vi "StartOnDemandAcquisitionRoutedMessage_Parse.vi"(8 "error in (no error)":errorcluster, 11 "message":variant) -> (0 "error out":errorcluster, 2 "on demand acq config":T1)   [LabVIEW 2017, in "EmsaAcquisition.lvlib"]
uses:
  <vilib>/addons/InsightCM/Devices/Shared/Emsa/EmsaAcquisition/EmsaAcquisition.lvlib
  <vilib>/addons/InsightCM/Devices/Shared/Emsa/EmsaAcquisition/controls/StartOnDemandAcquisitionRoutedMessage.ctl
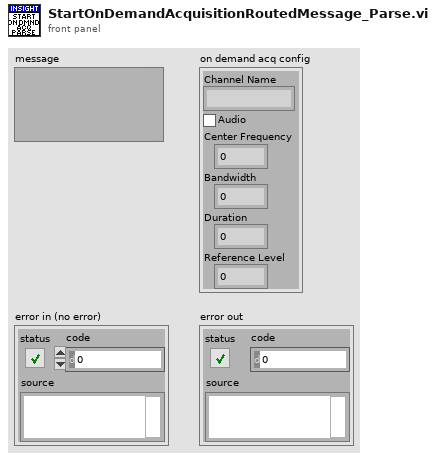
[diagram p1: front panel]
types:
  T1 = typedef "EmsaAcquisition.lvlib/StartOnDemandAcquisitionRoutedMessage.ctl" = cluster{"Channel Name":string, "Audio":bool, "Center Frequency":dbl, "Bandwidth":dbl, "Duration":dbl, "Reference Level":dbl}
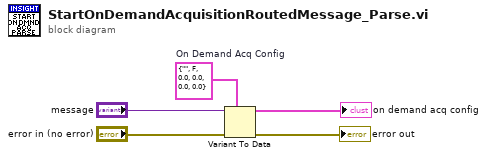
[diagram p0: block diagram]
diagram:
  w1 = T1 {"Channel Name"="", "Audio"=FALSE, "Center Frequency"=0.0, "Bandwidth"=0.0, "Duration"=0.0, "Reference Level"=0.0}  # On Demand Acq Config
  n1 = Variant To Data(error in="error in (no error)", type=w1, Variant="message") -> (data=→"on demand acq config":T1, error out=→"error out":errorcluster)
